vi "get channels.vi"(11 "EthernetIP configuration in":refnum<class "EthernetIP configuration.lvclass">) -> (2 "channels":refnum<class "TBM channel.lvclass">[](array[class]), 3 "EthernetIP configuration out":refnum<class "EthernetIP configuration.lvclass">)   [LabVIEW 2013, in "EthernetIP configuration.lvclass"]
uses:
  EthernetIP configuration.lvclass
  <vilib>/NI/Tag Bus Module Framework/channel/TBM channel.lvclass
  EthernetIP configuration.lvclass/EthernetIP configuration.ctl
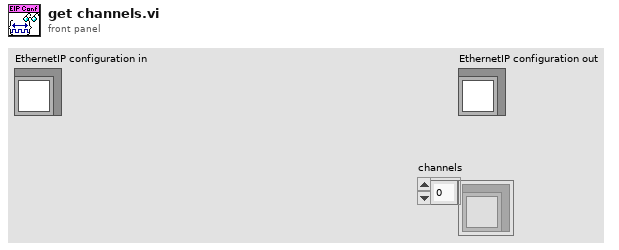
[diagram p1: front panel]
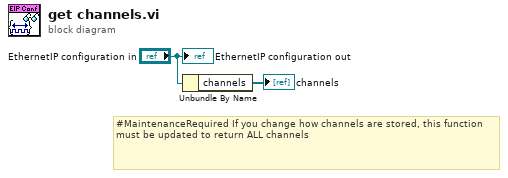
[diagram p0: block diagram]
diagram:
  # "#MaintenanceRequired If you change how channels are stored, this function must be updated to return ALL channels"
  n1 = Unbundle By Name("EthernetIP configuration in") -> ("channels"=→"channels":refnum<class "EthernetIP Channel.lvclass">[])
  "EthernetIP configuration out" <- "EthernetIP configuration in"
